vi "Ext.vi"(8 "error in (no error)":errorcluster, 9 "Val":variant, 10 "Tag":u16, 11 "Rigol DG822 UI in":refnum<class "Rigol DG822 UI.lvclass">) -> (0 "error out":errorcluster, 1 "Parsed":variant, 3 "Rigol DG822 UI out":refnum<class "Rigol DG822 UI.lvclass">)   [LabVIEW 2021, in "Rigol DG822 UI.lvlib" / "Rigol DG822 UI.lvclass"]
uses:
  Rigol DG822 UI.lvclass
  lib/controls.llb/RDG822ExtCall.ctl
  lib/controls.llb/AllWaveformDataCluster.ctl
  lib/controls.llb/DataCluster.ctl
  lib/controls.llb/FT Controls Cluster.ctl
  lib/controls.llb/String Indicators Cluster.ctl
  Rigol DG822 UI.lvclass/Rigol DG822 UI.ctl
  General/Files/lvlibp/Actors.lvlibp/Actors/Actors/Actors.lvclass
  D:/LabVIEW/General/Files/lvlibp/Actors.lvlibp/Actors/Actors/Actors.lvclass
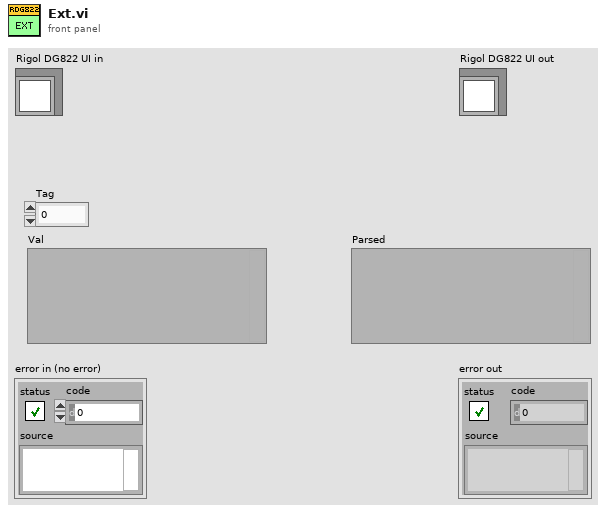
[diagram p1: front panel]
types:
  T1 = typedef "RDG822ExtCall.ctl" = enum16{"Get Data"}
  T2 = typedef "AllWaveformDataCluster.ctl" = cluster{"Data":T3, "F/T Ctrls":T4, "String Indcs":T5}
  T3 = typedef "DataCluster.ctl" = cluster{"Freq":cluster{"Freq":dbl, "FreqUnit":enum32{"No Selection", "MHz", "kHz", "Hz", "mHz", "uHz"}, "FreqUnitPrcs":dbl}, "Period":cluster{"Period":dbl, "PeriodUnit":enum32{"No Selection", "s", "ms", "us", "ns"}, "PeriodUnitPrcs":dbl}, "Ampl":cluster{"Ampl":dbl, "AmplUnit":enum32{"No Selection", "Vpp", "mVpp"}, "AmplUnitPrcs":dbl}, "HighL":cluster{"HighL":dbl, "HighLUnit":enum32{"No Selection", "V", "mV"}, "HighLUnitPrcs":dbl}, "Offset":cluster{"Offset":dbl, "OffsetUnit":enum32{"No Selection", "Vdc", "mVdc"}, "OffsetUnitPrcs":dbl}, "LowL":cluster{"LowL":dbl, "LowLUnit":enum32{"No Selection", "V", "mV"}, "LowLUnitPrcs":dbl}, "Phase":cluster{"Phase":dbl, "PhaseUnit":enum32{"°"}, "PhaseUnitPrcs":dbl}, "Duty":cluster{"Duty":dbl, "DutyUnit":enum32{"%"}, "DutyUnitPrcs":dbl}, "Width":cluster{"Width":dbl, "WidthUnit":enum32{"No Selection", "s", "ms", "us", "ns"}, "WidthUnitPrcs":dbl}, "RisEdge":cluster{"RisEdge":dbl, "RisEdgeUnit":enum32{"No Selection", "s", "ms", "us", "ns"}, "RisEdgeUnitPrcs":dbl}, "FallEdge":cluster{"FallEdge":dbl, "FallEdgeUnit":enum32{"No Selection", "s", "ms", "us", "ns"}, "FallEdgeUnitPrcs":dbl}}
  T4 = typedef "FT Controls Cluster.ctl" = cluster{"Freq/Period":bool, "Ampl/HighL":bool, "Offset/LowL":bool, "Duty/Width":bool}
  T5 = typedef "String Indicators Cluster.ctl" = cluster{"Freq-Period":string, "Ampl-HighL":string, "Offset-LowL":string, "Phase":string, "Duty-Width":string, "RisEdge":string, "FallEdge":string}
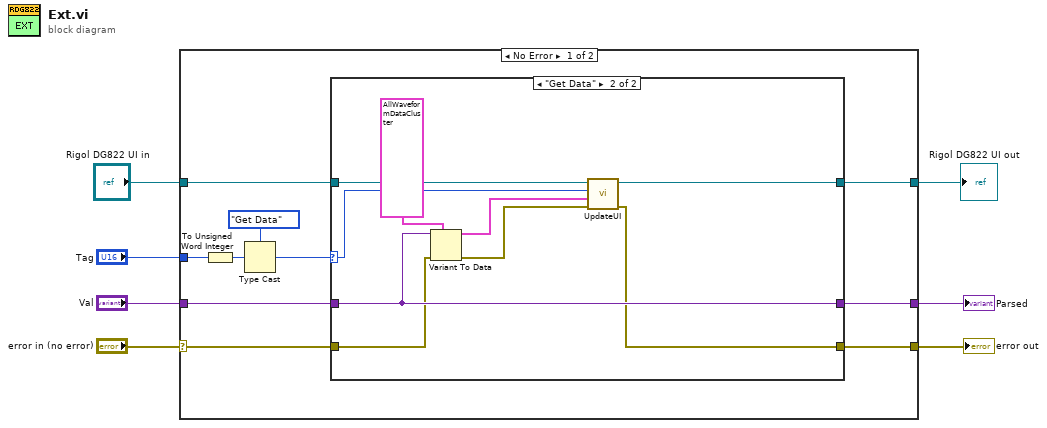
[diagram p0: block diagram]
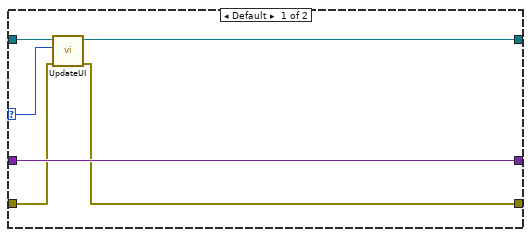
[diagram p2: hidden frame]
diagram:
  n1 = case shown="No Error" "error in (no error)" {
    selector: "error in (no error)" -> [w9 w34]
    tunnel: [w8 w34] -> w6
    tunnel: [w12 w33] -> w4
    tunnel: "Rigol DG822 UI in" -> [w13 w33]
    tunnel: "Tag" -> [w16 _]
    tunnel: "Val" -> [w15 _]
    tunnel: [w11 _] -> w1
    frame No Error {
      n2 = To Unsigned Word Integer(number=w16) -> (unsigned 16bit integer=w17:u16)
      n3 = Type Cast(type=RDG822ExtCall."Get Data", x=w17) -> (*(type *) &x=w14:T1)
      n4 = case shown="\"Get Data\"" w14 {
        selector: w14 -> [w22 w28]
        tunnel: w15 -> [w20 w32]
        tunnel: w13 -> [w23 w29]
        tunnel: [w21 w31] -> w12
        tunnel: [w20 w32] -> w11
        tunnel: w9 -> [w19 w27]
        tunnel: [w18 w25] -> w8
        frame Default {
          n5 = call "UpdateUI.vi"("error in (no error)"=w19, "Type"=w22, "Recursive in"=w23) -> ("error out"=w18:errorcluster, "Recursive out"=w21:refnum<class "Rigol DG822 UI.lvclass">)  [unwired: 7 in]
        }
        frame "Get Data" {
          n6 = Variant To Data(error in=w27, type=T2 {"Data"={"Freq"={"Freq"=1.0, "FreqUnit"=enum."kHz", "FreqUnitPrcs"=9.0}, "Period"={"Period"=1.0, "PeriodUnit"=enum."ms", "PeriodUnitPrcs"=7.0}, "Ampl"={"Ampl"=5.0, "AmplUnit"=enum."Vpp", "AmplUnitPrcs"=4.0}, "HighL"={"HighL"=2.5, "HighLUnit"=enum."V", "HighLUnitPrcs"=4.0}, "Offset"={"Offset"=0.0, "OffsetUnit"=enum."Vdc", "OffsetUnitPrcs"=4.0}, "LowL"={"LowL"=-2.5, "LowLUnit"=enum."V", "LowLUnitPrcs"=4.0}, "Phase"={"Phase"=0.0, "PhaseUnit"=enum."°", "PhaseUnitPrcs"=3.0}, "Duty"={"Duty"=50.0, "DutyUnit"=enum."%", "DutyUnitPrcs"=3.0}, "Width"={"Width"=500.0, "WidthUnit"=enum."us", "WidthUnitPrcs"=4.0}, "RisEdge"={"RisEdge"=10.0, "RisEdgeUnit"=enum."ns", "RisEdgeUnitPrcs"=1.0}, "FallEdge"={"FallEdge"=10.0, "FallEdgeUnit"=enum."ns", "FallEdgeUnitPrcs"=1.0}}, "F/T Ctrls"={"Freq/Period"=FALSE, "Ampl/HighL"=FALSE, "Offset/LowL"=FALSE, "Duty/Width"=FALSE}, "String Indcs"={"Freq-Period"="1.000,000,000 kHz", "Ampl-HighL"="5.000,0 Vpp", "Offset-LowL"="0.000,0 Vdc", "Phase"="0.000 °", "Duty-Width"="50.000 %", "RisEdge"="10.0 ns", "FallEdge"="10.0 ns"}} ("Params Data"), Variant=w32) -> (data=w30:T2, error out=w26:errorcluster)
          n7 = call "UpdateUI.vi"("error in (no error)"=w26, "Data"=w30, "Type"=w28, "Recursive in"=w29) -> ("error out"=w25:errorcluster, "Recursive out"=w31:refnum<class "Rigol DG822 UI.lvclass">)  [unwired: 6 in]
        }
      }
    }
    frame Error {
    }
  }
  "error out" <- w6
  "Rigol DG822 UI out" <- w4
  "Parsed" <- w1
